vi "切换k模式.vi"(8 "error in":errorcluster, 10 "切换K模式":enum16{"初始模式", "ByPassK"}(ring)) -> (0 "error out":errorcluster)   [LabVIEW 2016]
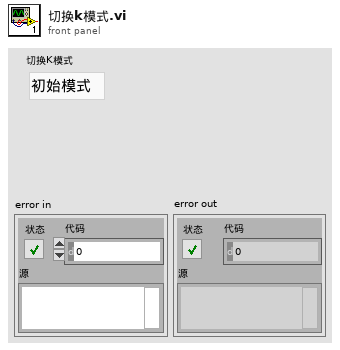
[diagram p1: front panel]
types:
  T1 = cluster{"byCmdType":u8, "bySubCmd":u8, "byPara":u8, "byAddr_h":u8, "byAddr_l":u8, "byAddr_ll":u8, "byLen_h":u8, "byLen_l":u8}
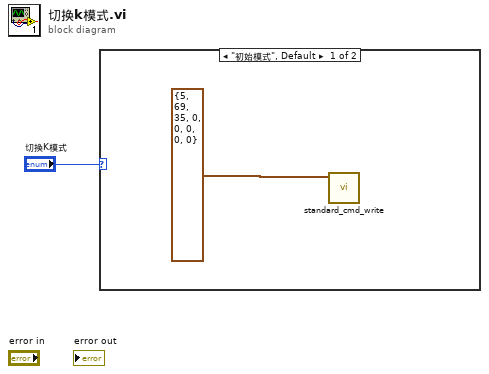
[diagram p0: block diagram]
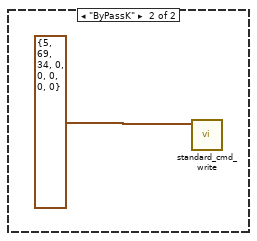
[diagram p2: hidden frame]
diagram:
  n1 = case shown="\"初始模式\", Default" "切换K模式" {
    frame "初始模式", Default {
      n2 = call "standard_cmd_write.vi"("cmd_std_header_t"=T1 {"byCmdType"=5, "bySubCmd"=69, "byPara"=35, "byAddr_h"=0, "byAddr_l"=0, "byAddr_ll"=0, "byLen_h"=0, "byLen_l"=0}) -> ()  [unwired: 10 in, 1 out]
    }
    frame "ByPassK" {
      n3 = call "standard_cmd_write.vi"("cmd_std_header_t"=T1 {"byCmdType"=5, "bySubCmd"=69, "byPara"=34, "byAddr_h"=0, "byAddr_l"=0, "byAddr_ll"=0, "byLen_h"=0, "byLen_l"=0}) -> ()  [unwired: 10 in, 1 out]
    }
  }
